vi "TestReport_main.vi"() -> ()   [LabVIEW 2016]
uses:
  TestReport_NumPoints.ctl
  TestReport_mods.ctl
panel:
  in  "Tipo":T1
  in  "Seção":string="01"
  out "Error out":errorcluster
  in  "Report path":path=path "L:/Documentos/00 SERVIÇOS/Tensão residual/São Sebastião - Osbat/Primeira e segunda seções/Relatorios/Seção 01"
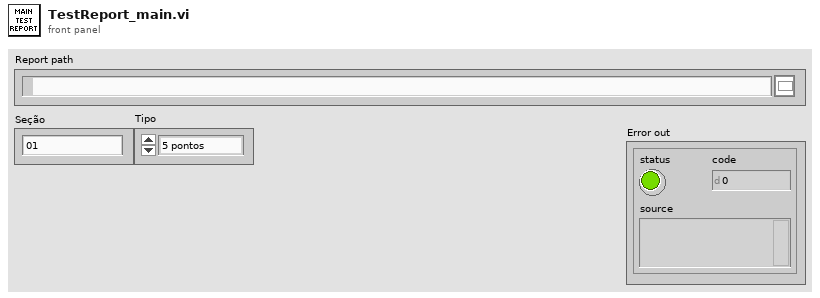
[diagram p1: front panel]
types:
  T1 = typedef "TestReport_NumPoints.ctl" = enum16{"5 pontos", "6 pontos"}
  T2 = typedef "TestReport_mods.ctl" = enum16{"Open", "Table", "Image", "Tag", "ResizeAll", "Close"}
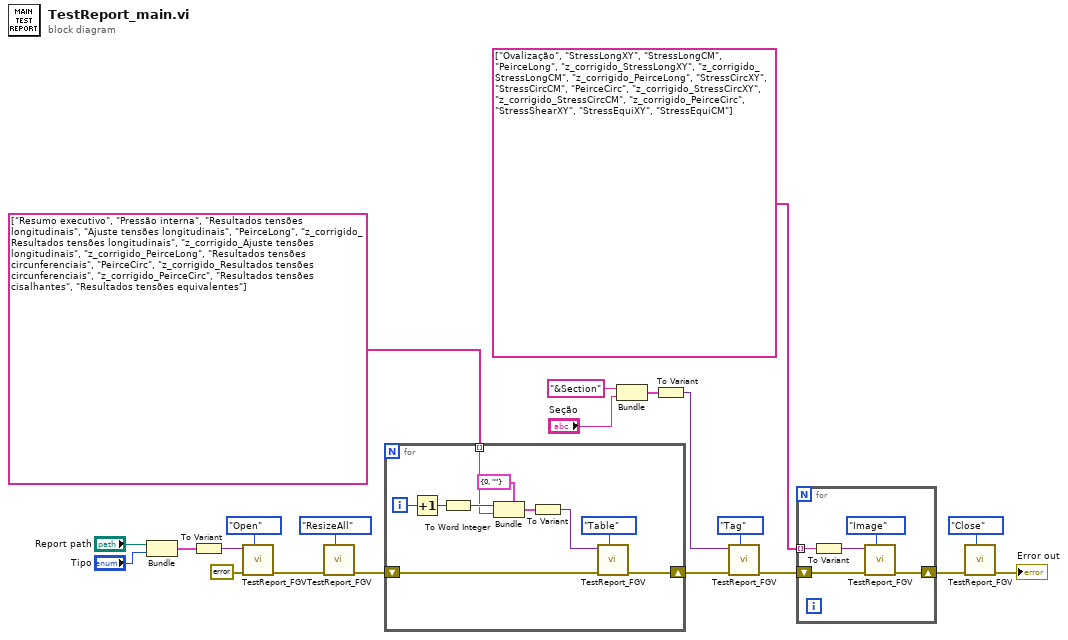
[diagram p0: block diagram]
diagram:
  n1 = Bundle("Report path"="Report path", "Tipo"="Tipo") -> (w1:cluster{"Report path":path, "Tipo":T1})  [unwired: 1 in]
  n2 = To Variant(anything=w1) -> (Variant=w19:variant)
  n3 = call "TestReport_FGV.vi"("ModReport"=TestReport_mods."Open", "Error in"=errorcluster {"status"=FALSE, "code"=0, "source"=""}, "Parameter"=w19) -> ("Error out"=w8:errorcluster)  [unwired: 8 in]
  n4 = call "TestReport_FGV.vi"("ModReport"=TestReport_mods."ResizeAll", "Error in"=w8) -> ("Error out"=w7:errorcluster)  [unwired: 9 in]
  n5 = for {
    tunnel: string[] ["Resumo executivo", "Pressão interna", "Resultados tensões longitudinais", "Ajuste tensões longitudinais", "PeirceLong", "z_corrigido_Resultados tensões longitudinais", "z_corrigido_Ajuste tensões longitudinais", "z_corrigido_PeirceLong", "Resultados tensões circunferenciais", "PeirceCirc", "z_corrigido_Resultados tensões circunferenciais", "z_corrigido_PeirceCirc", "Resultados tensões cisalhantes", "Resultados tensões equivalentes"] ("Name") -> [w22] mode=indexing
    shift-right: [w25] -> w16
    shift-left: w7 -> [w28]
    i -> [w27]
    n6 = Increment(x=w27) -> (x+1=w26:i32)
    n7 = To Word Integer(number=w26) -> (16bit integer=w23:i16)
    n8 = Bundle(cluster=cluster{i16, string} {0, ""}, w23, w22) -> (w30:cluster{i16, string})
    n9 = To Variant(anything=w30) -> (Variant=w31:variant)
    n10 = call "TestReport_FGV.vi"("ModReport"=TestReport_mods."Table", "Error in"=w28, "Parameter"=w31) -> ("Error out"=w25:errorcluster)  [unwired: 8 in]
  }
  n11 = Bundle("Name"="&Section", "Seção"="Seção") -> (w13:cluster{"Name":string, "Seção":string})  [unwired: 1 in]
  n12 = To Variant(anything=w13) -> (Variant=w12:variant)
  n13 = call "TestReport_FGV.vi"("ModReport"=TestReport_mods."Tag", "Error in"=w16, "Parameter"=w12) -> ("Error out"=w11:errorcluster)  [unwired: 8 in]
  n14 = for {
    tunnel: string[] ["Ovalização", "StressLongXY", "StressLongCM", "PeirceLong", "z_corrigido_StressLongXY", "z_corrigido_StressLongCM", "z_corrigido_PeirceLong", "StressCircXY", "StressCircCM", "PeirceCirc", "z_corrigido_StressCircXY", "z_corrigido_StressCircCM", "z_corrigido_PeirceCirc", "StressShearXY", "StressEquiXY", "StressEquiCM"] ("Name") -> [w34] mode=indexing
    shift-right: [w32] -> w5
    shift-left: w11 -> [w35]
    n15 = To Variant(anything=w34) -> (Variant=w33:variant)
    n16 = call "TestReport_FGV.vi"("ModReport"=TestReport_mods."Image", "Error in"=w35, "Parameter"=w33) -> ("Error out"=w32:errorcluster)  [unwired: 8 in]
  }
  n17 = call "TestReport_FGV.vi"("ModReport"=TestReport_mods."Close", "Error in"=w5) -> ("Error out"=→"Error out":errorcluster)  [unwired: 9 in]
